vi "Where I Am.vi"   [LabVIEW 2010]
uses:
  5.0-Global.vi
types:
  T1 = cluster{"X (Current)":dbl, "Y (Current) ":dbl, "Heading":dbl, "Steering Angle":dbl}
  T2 = typedef "MDFArray.ctl" = T3[]
  T3 = typedef "MissionDefinitionFile.ctl" = cluster{"Waypoint #":dbl, "X (waypoint)":dbl, "Y (waypoint)":dbl, "Vel (desired)":dbl, "Dwell Time":dbl, "Behavior":enum16{"OpenFieldTransit", "WallFollow", "LaneFollow", "ManualMode"}, "Expand1":dbl, "Expand2":dbl, "Expand3":dbl}
  T4 = typedef "3.2-Where Sensor Typedef.ctl" = cluster{"4.2.2-GPS Data":T5, "4.2.1-VectorNav Data":T6, "4.2.1-VectorNav Status":string}
  T5 = typedef "Current GPS Data.ctl" = cluster{"Lattitude (dd.mmmmmm)":dbl, "Longitude (dd.mmmmmm)":dbl, "EST Time":timestamp}
  T6 = typedef "3.2.1-VectorNav Data.ctl" = cluster{"Yaw":dbl, "Pitch":dbl, "Roll":dbl}
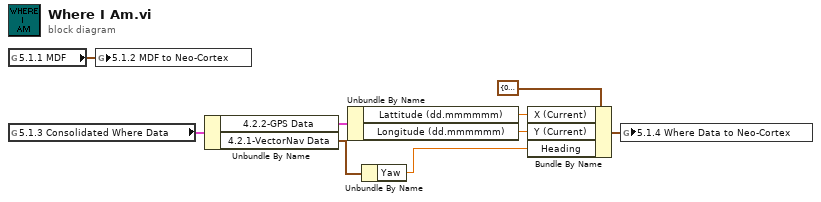
[diagram p0: block diagram]
diagram:
  n1 = global read "5.0-Global.vi" "5.1.1 MDF"() -> (w8:T2)
  n2 = global read "5.0-Global.vi" "5.1.3 Consolidated Where Data"() -> (w9:T4)
  n3 = global write "5.0-Global.vi" "5.1.2 MDF to Neo-Cortex"(w8) -> ()
  n4 = Unbundle By Name(w9) -> ("4.2.2-GPS Data"=w7:T5, "4.2.1-VectorNav Data"=w2:T6)
  n5 = Unbundle By Name(w7) -> ("Lattitude (dd.mmmmmm)"=w6:dbl, "Longitude (dd.mmmmmm)"=w5:dbl)
  n6 = Unbundle By Name(w2) -> ("Yaw"=w1:dbl)
  n7 = Bundle By Name(cluster=T1 {"X (Current)"=0.0, "Y (Current) "=0.0, "Heading"=0.0, "Steering Angle"=0.0} ("5.1.4 Where Data to Neo-Cortex"), "X (Current)"=w6, "Y (Current)"=w5, "Heading"=w1) -> (w3:T1)
  n8 = global write "5.0-Global.vi" "5.1.4 Where Data to Neo-Cortex"(w3) -> ()
